vi "FdxCmdTMSetSubscriberCvi.vi"(8 "error in":errorcluster, 9 "TMSetSubscriberIn":T1, 10 "TMHandle":u32, 11 "InstrumentHandle":u32) -> (0 "error out":errorcluster, 2 "TMHandleOut":u32, 3 "InstrumentHandle":u32)   [LabVIEW 2020, in "AIM664LV.lvlib"]
doc: "This function is used to set up a Time Manager for communication with a subscriber. This function can not be called once a Time Manager has been started."
uses:
  AIM664LV.lvlib
  AFDX_LibraryAdmin/FdxGlobalDllPath.vi
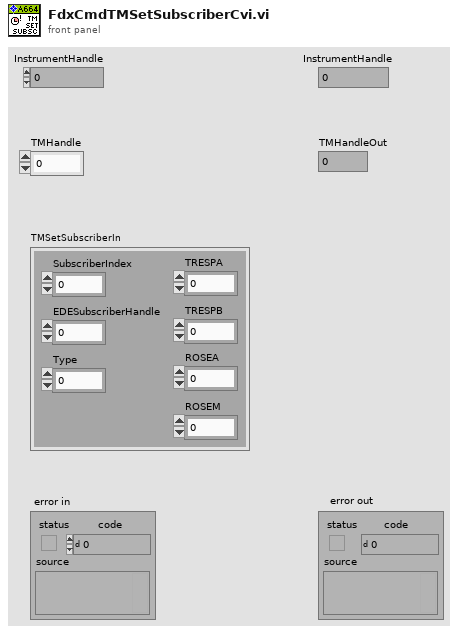
[diagram p1: front panel]
types:
  T1 = cluster{"SubscriberIndex":u8, "EDESubscriberHandle":u32, "Type":u32, "TRESPA":u32, "TRESPB":u32, "ROSEA":u16, "ROSEM":u16}
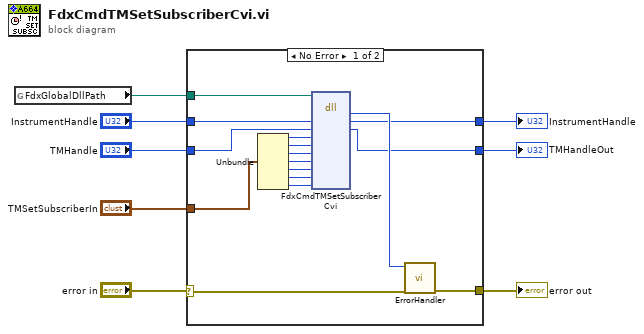
[diagram p0: block diagram]
diagram:
  n1 = global read "FdxGlobalDllPath.vi" "FdxGlobalDllPath"() -> (w6:path)
  n2 = case shown="No Error" "error in" {
    selector: "error in" -> [w23 w27]
    tunnel: [w24 w27] -> w8
    tunnel: w6 -> [w14 _]
    tunnel: "InstrumentHandle" -> [w13 w26]
    tunnel: [w12 w26] -> w4
    tunnel: "TMHandle" -> [w11 w25]
    tunnel: "TMSetSubscriberIn" -> [w10 _]
    tunnel: [w9 w25] -> w1
    frame No Error {
      n3 = Unbundle(w10) -> ("SubscriberIndex"=w21:u8, "EDESubscriberHandle"=w20:u32, "Type"=w19:u32, "TRESPA"=w18:u32, "TRESPB"=w17:u32, "ROSEA"=w16:u16, "ROSEM"=w15:u16)
      n4 = dll-call lib="aim_fdx.19.dll" fn="FdxCmdTMSetSubscriberCvi"(path in=w14, "InstrumentHandle"=w13, "TMHandle"=w11, "SubscriberIndex"=w21, "EDESubscriberHandle"=w20, "Type"=w19, "TRESPA"=w18, "TRESPB"=w17, "ROSEA"=w16, "ROSEM"=w15) -> ("status"=w22:i32, "InstrumentHandle"=w12:u32, "TMHandle"=w9:u32)  [unwired: 9 in, 2 out]
      n5 = call "ErrorHandler.vi"("error in"=w23, "AIM Error"=w22) -> ("error out"=w24:errorcluster)  [unwired: 9 in]
    }
    frame Error {
    }
  }
  "error out" <- w8
  "InstrumentHandle" <- w4
  "TMHandleOut" <- w1
